vi "Final.vi"() -> ()   [LabVIEW 2016]
uses:
  <vilib>/measure/matone.llb/Extract Single Tone Information N Chan.vi
  <vilib>/addons/control/pid/pid.llb/PID (DBL).vi
  <vilib>/measure/NI_MAPro.lvlib
  <vilib>/addons/control/pid/NI_PID_pid.lvlib
  <vilib>/ptbypt/NI_PtbyPt.lvlib
panel:
  out "Frequency":dbl(graph)=0.22472733409108478
  in  "Synchronize":bool
  in  "Short Circuit":bool
  out "Torque (N*m)":dbl=0.22472733409108478 format="%0.2f"
  in  "stop (F)":bool caption="Stop (F)"
  out "Out Amplitude (A)":dbl[](array[numeric])=[0.025244298013845933, 0.025633108860585403, 0.037271732325756333] format="%.2p"
  out "DAQ Buck PID (V)":dbl=3.842235019393467
  in  "Amplitude PID % Range":cluster{"output high":dbl, "output low":dbl}={"output high"=-2.0, "output low"=-6.0} {"output low" format="%.2f"; "output high" format="%.2f"}
  in  "Amplitude PID Gains":T1={"proportional gain (Kc)"=0.01, "integral time (Ti, min)"=0.01, "derivative time (Td, min)"=0.0} {"derivative time (Td, min)" format="%.3f"; "integral time (Ti, min)" format="%.3f"; "proportional gain (Kc)" format="%.3f"}
  in  "Set Amplitude (V)":dbl=172.5 format="%.2f"
  in  "Contactor On":bool
  out "DCX (V)":dbl=2.29892646799261 format="%.2f"
  in  "Frequency PID gains":T1={"proportional gain (Kc)"=0.04, "integral time (Ti, min)"=0.025, "derivative time (Td, min)"=0.0} {"derivative time (Td, min)" format="%.3f"; "integral time (Ti, min)" format="%.3f"; "proportional gain (Kc)" format="%.3f"}
  out "Speed Frequency (Hz)":dbl=59.88103434746426
  in  "Frequency PID Output Range":cluster{"output high":dbl, "output low":dbl}={"output high"=3.0, "output low"=0.0} {"output low" format="%.2f"; "output high" format="%.2f"}
  in  "Set Frequency (Hz)":dbl=60.0 format="%.2f"
  out "Out Waveform (V)":dynamicdata(graph)=[{"t0"=timestamp(3574869668.903589 s since 1904-01-01), "dt"=0.00019999999999999998, "Y"=array[1500 elements], "attributes"=variant("NI_ChannelName"=variant(string "Wave 1"), "NI_UnitDescription"=variant(string "Volts"))}, {"t0"=timestamp(3574869668.903639 s since 1904-01-01), "dt"=0.00019999999999999998, "Y"=array[1500 elements], "attributes"=variant("NI_ChannelName"=variant(string "Wave 2"), "NI_UnitDescription"=variant(string "Volts"))}, {"t0"=timestamp(3574869668.903689 s since 1904-01-01), "dt"=0.00019999999999999998, "Y"=array[1500 elements], "attributes"=variant("NI_ChannelName"=variant(string "Wave 3"), "NI_UnitDescription"=variant(string "Volts"))}, {"t0"=timestamp(3574869668.903739 s since 1904-01-01), "dt"=0.00019999999999999998, "Y"=array[1500 elements], "attributes"=variant("NI_ChannelName"=variant(string "Speed Sensor"), "NI_UnitDescription"=variant(string "Volts"))}] caption="Voltage Waveforms"
  out "Out Frequency (Hz)":dbl[](array[numeric])=[59.88320535202167, 59.8834300081703, 59.883241381328794, 1796.4310304239277] format="%.2p"
  out "Out Amplitude (V) Pk-0":dbl[](array[numeric])=[165.06811998763195, 175.51934446413858, 169.11250287517208, 2.7646731644509277] format="%.2p"
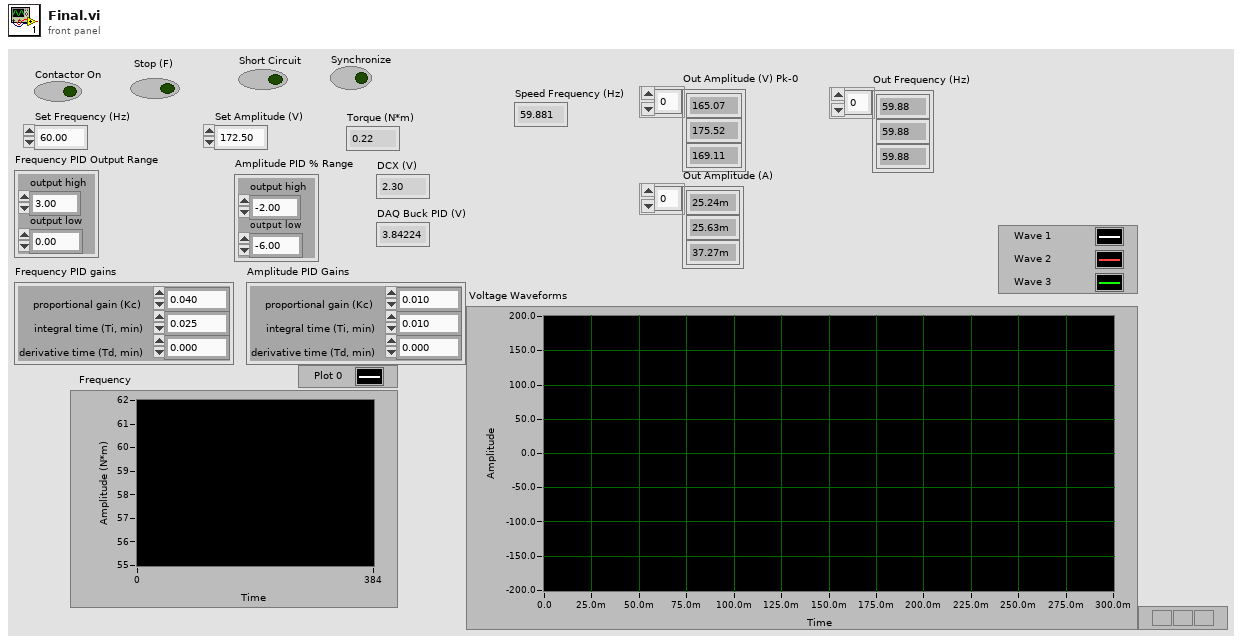
[diagram p1: front panel]
types:
  T1 = cluster{"proportional gain (Kc)":dbl, "integral time (Ti, min)":dbl, "derivative time (Td, min)":dbl}
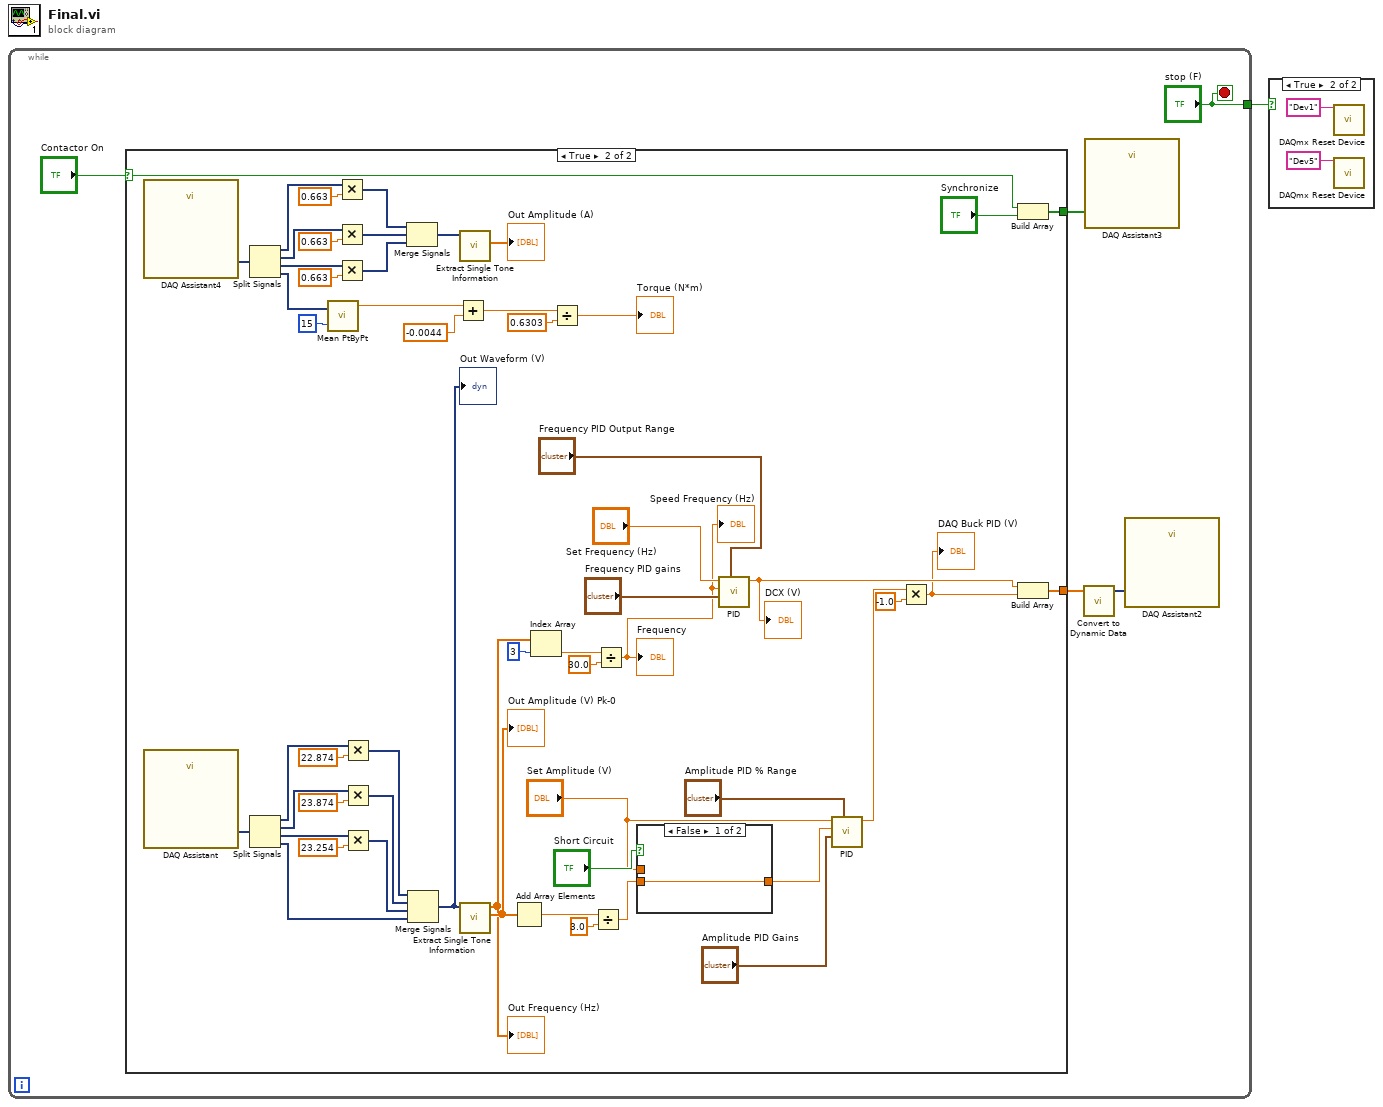
[diagram p0: block diagram]
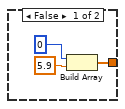
[diagram p3: hidden frame]
diagram:
  n1 = while {
    tunnel: ["stop (F)"] -> w1
    stop <- "stop (F)" stop-if-true
    n2 = case shown="True" "Contactor On" {
      selector: "Contactor On" -> [_ w62]
      tunnel: [w7 w65] -> w6
      tunnel: [_ w61] -> w4
      frame False {
        n3 = Build Array(0, 5.9) -> (w7:dbl[])
      }
      frame True {
        n4 = call "DAQ Assistant4"() -> ("data"=w45:dynamicdata)  [unwired: 16 in, 3 out]
        n5 = call "DAQ Assistant"() -> ("data"=w49:dynamicdata)  [unwired: 16 in, 3 out]
        n6 = Split Signals(w45) -> (w44:dynamicdata, w43:dynamicdata, w42:dynamicdata, w10:dynamicdata)  [unwired: 4 in]
        n7 = Split Signals(w49) -> (w40:dynamicdata, w38:dynamicdata, w36:dynamicdata, w31:dynamicdata)  [unwired: 4 in]
        n8 = call <vilib>:"Mean PtByPt.vi"("x"=w10, "sample length"=15) -> ("mean"=w54:dbl)  [unwired: 2 in, 1 out]
        n9 = Multiply(x=w44, y=0.663) -> (x*y=w14:dynamicdata)
        n10 = Multiply(x=w43, y=0.663) -> (x*y=w25:dynamicdata)
        n11 = Multiply(x=w42, y=0.663) -> (x*y=w27:dynamicdata)
        n12 = Multiply(x=w40, y=22.874) -> (x*y=w28:dynamicdata)
        n13 = Multiply(x=w38, y=23.874) -> (x*y=w26:dynamicdata)
        n14 = Multiply(x=w36, y=23.254) -> (x*y=w24:dynamicdata)
        n15 = Merge Signals(w14, w25, w27) -> (w29:dynamicdata)
        n16 = Merge Signals(w28, w26, w24, w31) -> (w35:dynamicdata)
        "Out Waveform (V)" <- w35
        n17 = Add(x=w54, y=-0.0044) -> (x+y=w52:dbl)
        n18 = call-poly <vilib>:"Extract Single Tone Information.vi"("time signals in"=w29) -> ("detected amplitudes"=→"Out Amplitude (A)":dbl[])  [unwired: 5 in, 5 out]
        n19 = call-poly <vilib>:"Extract Single Tone Information.vi"("time signals in"=w35) -> ("detected amplitudes"=w32:dbl[], "detected frequencies"=w30:dbl[])  [unwired: 5 in, 4 out]
        "Out Amplitude (V) Pk-0" <- w32
        "Out Frequency (Hz)" <- w30
        n20 = Add Array Elements(numeric array=w32) -> (sum=w60:dbl)
        n21 = Index Array(array=w30, index=3) -> (element=w33:dbl)
        n22 = Divide(x=w52, y=0.6303) -> (x/y=→"Torque (N*m)":dbl)
        n23 = Divide(x=w60, y=3.0) -> (x/y=w20:dbl)
        n24 = Divide(x=w33, y=30.0) -> (x/y=w12:dbl)
        "Speed Frequency (Hz)" <- w12
        "Frequency" <- w12
        n25 = case shown="False" "Short Circuit" {
          tunnel: w20 -> [w66 _]
          tunnel: [w66 w67] -> w11
          tunnel: "Set Amplitude (V)" -> [_ w67]
          frame False {
          }
          frame True {
          }
        }
        n26 = call-poly <vilib>:"PID.vi"("output range"="Frequency PID Output Range", "PID gains"="Frequency PID gains", "process variable"=w12, "setpoint"="Set Frequency (Hz)") -> ("output"=w22:dbl)  [unwired: 6 in, 1 out]
        "DCX (V)" <- w22
        n27 = call-poly <vilib>:"PID.vi"("output range"="Amplitude PID % Range", "PID gains"="Amplitude PID Gains", "process variable"=w11, "setpoint"="Set Amplitude (V)") -> ("output"=w17:dbl)  [unwired: 6 in, 1 out]
        n28 = Multiply(x=w17, y=-1.0) -> (x*y=w16:dbl)
        "DAQ Buck PID (V)" <- w16
        n29 = Build Array(w62, "Synchronize") -> (w61:bool[])
        n30 = Build Array(w22, w16) -> (w65:dbl[])
      }
    }
    n31 = call "Convert to Dynamic Data"("Array"=w6) -> ("Dynamic Data Type"=w5:dynamicdata)  [unwired: 3 in]
    n32 = call "DAQ Assistant3"("data"=w4) -> ()  [unwired: 17 in, 2 out]
    n33 = call "DAQ Assistant2"("data"=w5) -> ()  [unwired: 17 in, 2 out]
  }
  n34 = case shown="True" w1 {
    frame False {
    }
    frame True {
      n35 = call <vilib>:"DAQmx Reset Device.vi"("device in"="Dev1" ("y")) -> ()  [unwired: 14 in, 1 out]
      n36 = call <vilib>:"DAQmx Reset Device.vi"("device in"="Dev5" ("y")) -> ()  [unwired: 14 in, 1 out]
    }
  }
